vi "connectSubDataSubscribe.vi"(8 "error in (no error)":errorcluster, 11 "MiddlewareSALThisComponent in":refnum<class "MiddlewareSALThisComponent.lvclass">) -> (0 "error out":errorcluster, 3 "MiddlewareSALThisComponent out":refnum<class "MiddlewareSALThisComponent.lvclass">)   [LabVIEW 2016, in "MiddlewareSALThisComponent.lvclass"]
uses:
  MiddlewareSALThisComponent.lvclass
  ProgrammaticInitialization/ProgrammaticInitialization.lvclass
  ts_sallv_sedspectrometer/SALLV_sedSpectrometer.lvlib
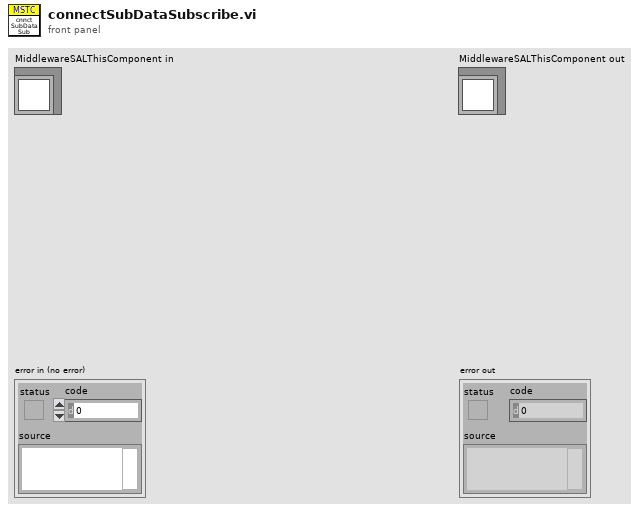
[diagram p1: front panel]
types:
  T1 = typedef "ProgrammaticInitialization.lvclass/cmdsToSubscribeDL.ctl" = string[]
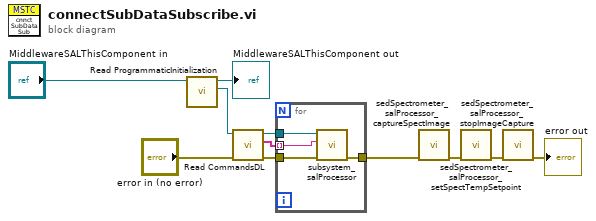
[diagram p0: block diagram]
diagram:
  n1 = call-dynamic "Read ProgrammaticInitialization.vi"("MiddlewareSALThisComponent in"="MiddlewareSALThisComponent in") -> ("ProgrammaticInitialization"=w10:refnum<class "ProgrammaticInitialization.lvclass">, "MiddlewareSALThisComponent out"=→"MiddlewareSALThisComponent out":refnum<class "MiddlewareSALThisComponent.lvclass">)  [unwired: 8 in, 1 out]
  n2 = call-dynamic "Read CommandsDL.vi"("error in (no error)"="error in (no error)", "ProgrammaticInitialization in"=w10) -> ("error out"=w5:errorcluster, "CommandsDL"=w8:T1, "ProgrammaticInitialization out"=w7:refnum<class "ProgrammaticInitialization.lvclass">)  [unwired: 7 in]
  n3 = for {
    tunnel: w8 -> [w15] mode=indexing
    tunnel: w7 -> [w14]
    tunnel: w5 -> [w13]
    tunnel: [w12] -> w2
    n4 = call "subsystem_salProcessor.vi"("error in (no error)"=w13, "topic"=w15, "ProgrammaticInitialization in"=w14) -> ("error out"=w12:errorcluster)  [unwired: 7 in, 1 out]
  }
  n5 = call "sedSpectrometer_salProcessor_captureSpectImage.vi"("error in (no error)"=w2) -> ("error out"=w3:errorcluster)  [unwired: 9 in, 1 out]
  n6 = call "sedSpectrometer_salProcessor_setSpectTempSetpoint.vi"("error in (no error)"=w3) -> ("error out"=w4:errorcluster)  [unwired: 9 in, 1 out]
  n7 = call "sedSpectrometer_salProcessor_stopImageCapture.vi"("error in (no error)"=w4) -> ("error out"=→"error out":errorcluster)  [unwired: 9 in, 1 out]
